vi "Write to RF Synth Bd1 Only.vi"(0 "Address Byte":u8, 2 "BD 1 Byte":u8) -> ()   [LabVIEW 2014]
uses:
  <vilib>/Platform/TimedLoop/XDataNode/timing_clust.ctl
  <vilib>/Platform/TimedLoop/XDataNode/nitl_modes.ctl
  <vilib>/Platform/TimedLoop/XDataNode/wakeup.ctl
  <vilib>/rvi/Emulation/niFpgaSctlEmulationGetInTimedLoop.vi
  <vilib>/rvi/Emulation/niFpgaEmulationReportErrorSimple.vi
  <vilib>/rvi/Emulation/niFpgaGetClockAttributes.vi
  <vilib>/rvi/Emulation/niFpgaCriticalErrorInLSC.vi
  <vilib>/rvi/eio/common/nirviEmuTemplateMethod_errors.vi
  <vilib>/Platform/TimedLoop/XDataNode/XDataNode.xnode
  <vilib>/eio/EIONode/EIONode.xnode
  <vilib>/Platform/TimedLoop/XDataNode/XDNodeRunTimeDep.lvlib
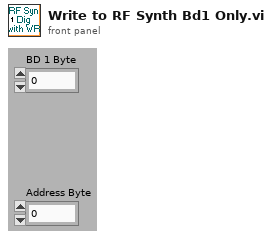
[diagram p1: front panel]
types:
  T1 = typedef "XDNodeRunTimeDep.lvlib/timing_clust.ctl" = cluster{"Expected End [f-1]":u64, "Actual End [f-1]":u64, "Finished Late? [f-1]":bool, "Expected End [i-1]":u64, "Actual End [i-1]":u64, "Finished Late? [i-1]":bool, "Expected Start [i]":u64, "Actual Start [i]":u64, "Expected Start [f]":u64, "Actual Start [f]":u64, "Source Name":string, "Structure Name":string, "Period":i64, "Deadline":i64, "Offset":i64, "Start":i64, "Priority":i32, "Timeout":i32, "Mode":T2, "Wakeup Reason":T3, "Error":errorcluster, "Source Type":string, "Secondary Source Type":string, "Global End Time":u64, "Global Start Time":u64, "Frame Duration":u64, "Iteration Duration":u64, "Assigned CPU":i32, "I/O Scan Engine Mode":u32}
  T2 = typedef "XDNodeRunTimeDep.lvlib/nitl_modes.ctl" = enum32{"No Change", "Process missed periods, maintain original phase", "Discard missed periods, maintain original phase", "Process missed periods, ignore original phase", "Discard missed periods, ignore original phase"}
  T3 = typedef "XDNodeRunTimeDep.lvlib/wakeup.ctl" = enum32{"Normal", "Aborted", "Asynchronous wakeup", "Timing source error", "Timed loop error", "Timeout"}
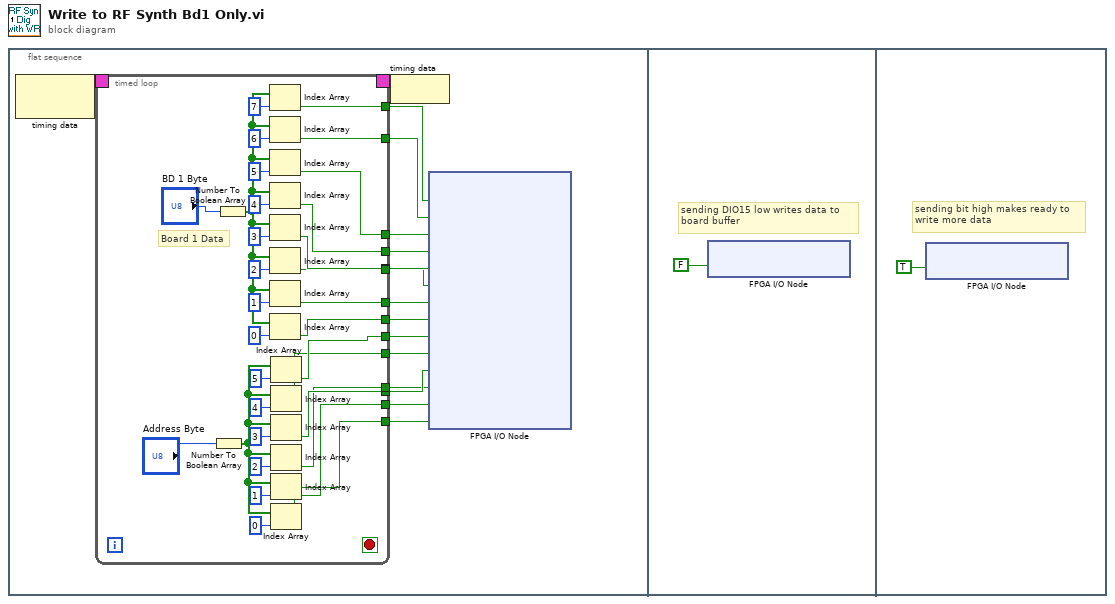
[diagram p0: block diagram]
diagram:
  n1 = flat-sequence {
    frame #0 {
      n2 = node-c288() -> (w2:T1)  [unwired: 1 in]
      n3 = timed-loop {
        timing: w2 -> [_]
        timing-out: [_] -> w1
        tunnel: [w32] -> w16
        tunnel: [w31] -> w15
        tunnel: [w30] -> w14
        tunnel: [w29] -> w13
        tunnel: [w28] -> w12
        tunnel: [w27] -> w11
        tunnel: [w26] -> w10
        tunnel: [w25] -> w9
        tunnel: [w24] -> w8
        tunnel: [w23] -> w7
        tunnel: [w22] -> w6
        tunnel: [w21] -> w5
        tunnel: [w20] -> w4
        tunnel: [w19] -> w3
        stop <- _ stop-if-true
        # "Board 1 Data"
        n4 = Number To Boolean Array(number="Address Byte") -> (Boolean array=w47:bool[])
        n5 = Number To Boolean Array(number="BD 1 Byte") -> (Boolean array=w48:bool[])
        n6 = Index Array(array=w48, index=7) -> (element=w32:bool)
        n7 = Index Array(array=w48, index=6) -> (element=w31:bool)
        n8 = Index Array(array=w48, index=5) -> (element=w30:bool)
        n9 = Index Array(array=w48, index=4) -> (element=w29:bool)
        n10 = Index Array(array=w48, index=3) -> (element=w28:bool)
        n11 = Index Array(array=w48, index=2) -> (element=w27:bool)
        n12 = Index Array(array=w48, index=1) -> (element=w26:bool)
        n13 = Index Array(array=w48, index=0) -> (element=w25:bool)
        n14 = Index Array(array=w47, index=5) -> (element=w24:bool)
        n15 = Index Array(array=w47, index=4) -> (element=w23:bool)
        n16 = Index Array(array=w47, index=3) -> (element=w22:bool)
        n17 = Index Array(array=w47, index=2) -> (element=w21:bool)
        n18 = Index Array(array=w47, index=1) -> (element=w20:bool)
        n19 = Index Array(array=w47, index=0) -> (element=w19:bool)
      }
      n20 = node-c288(w1) -> ()
      n21 = xnode "FPGA I/O Node"("Connector1/DIO0"=w16, "Connector1/DIO1"=w15, "Connector1/DIO2"=w14, "Connector1/DIO3"=w13, "Connector1/DIO4"=w12, "Connector1/DIO5"=w11, "Connector1/DIO6"=w10, "Connector1/DIO7"=w9, "Connector1/DIO8"=w8, "Connector1/DIO9"=w7, "Connector1/DIO10"=w6, "Connector1/DIO11"=w5, "Connector1/DIO12"=w4, "Connector1/DIO13"=w3) -> ()  [unwired: 14 in, 14 out]
    }
    frame #1 {
      # "sending DIO15 low writes data to \nboard buffer"
      n22 = xnode "FPGA I/O Node"("Connector1/DIO15"=FALSE) -> ()  [unwired: 1 in, 1 out]
    }
    frame #2 {
      # "sending bit high makes ready to\nwrite more data"
      n23 = xnode "FPGA I/O Node"("Connector1/DIO15"=TRUE) -> ()  [unwired: 1 in, 1 out]
    }
  }
